vi "Configure Channel (TC Delta).vi"(0 "VISA resource name":refnum<visa-resource-name>, 1 "Reference Channel (0001)":string="0001", 5 "Channel (0001)":string="0001", 7 "Enable Channel (True)":bool=TRUE, 9 "Range and Span":T1={"Thermocouple Type (0 : R)"=0, "Enable Span (False)"=FALSE, "Lower Span (0.0)"=0.0, "Upper Span (1760.0)"=1760.0, "Bias (0)"=0.0} {"Thermocouple Type (0 : R)" items=["R", "S", "B", "K", "K-H", "E", "J", "T", "N", "W", "L", "U", "WRe3-25", "PLATINEL", "PR40-20", "KpvsAu7Fe", "NiNiMo", "WWRe26", "N14", "XK"]; "Bias (0)" min=-99999.9 max=99999.9 format="%.1f"; "Upper Span (1760.0)" min=-10000.0 max=10000.0 format="%#.1f"; "Lower Span (0.0)" min=-10000.0 max=10000.0 format="%#.1f"}, 11 "error in (no error)":errorcluster) -> (4 "VISA resource name out":refnum<visa-resource-name>, 6 "Channel":string, 15 "error out":errorcluster)   [LabVIEW 2020, in "Yokogawa GX Series.lvlib"]
doc: "Sets the input range as thermocouple.\n\nCommand: SRangeAI"
uses:
  <instrlib>/Yokogawa GX Series/Yokogawa GX Series.lvlib
  <instrlib>/Yokogawa GX Series/Private/TC Range.vi
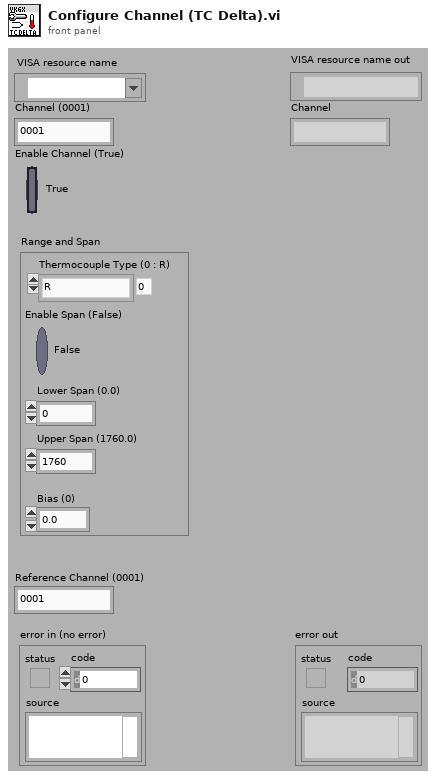
[diagram p1: front panel]
types:
  T1 = cluster{"Thermocouple Type (0 : R)":i32, "Enable Span (False)":bool, "Lower Span (0.0)":dbl, "Upper Span (1760.0)":dbl, "Bias (0)":dbl}
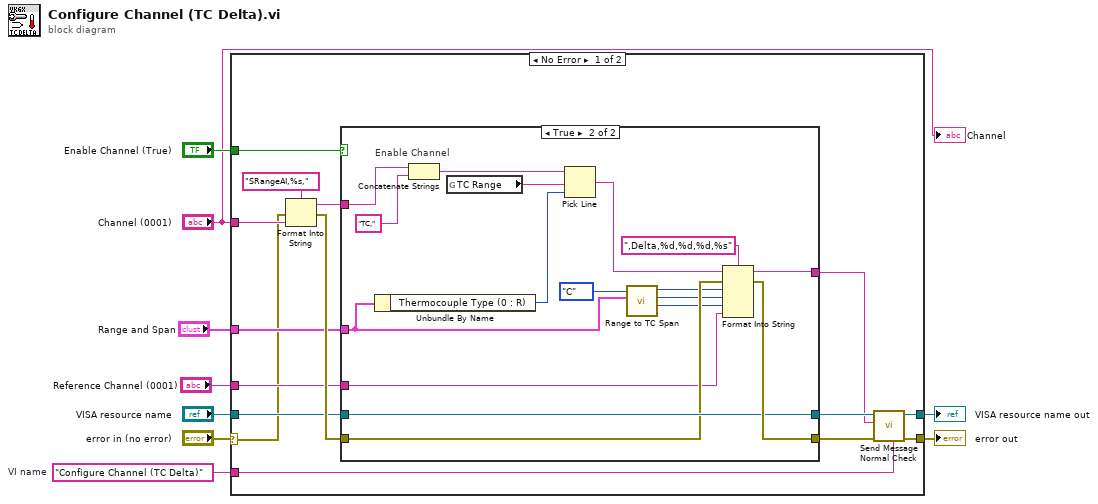
[diagram p0: block diagram]
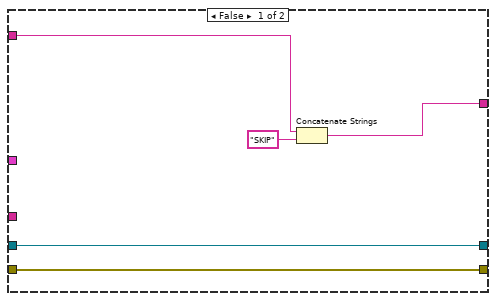
[diagram p2: hidden frame]
diagram:
  w4 = "Configure Channel (TC Delta)"  # VI name
  n1 = case shown="No Error" "error in (no error)" {
    selector: "error in (no error)" -> [w10 w47]
    tunnel: "Enable Channel (True)" -> [w21 _]
    tunnel: "VISA resource name" -> [w20 w48]
    tunnel: "Range and Span" -> [w19 _]
    tunnel: [w16 w48] -> w6
    tunnel: [w15 w47] -> w5
    tunnel: w4 -> [w14 _]
    tunnel: "Reference Channel (0001)" -> [w12 _]
    tunnel: "Channel (0001)" -> [w11 _]
    frame No Error {
      n2 = Format Into String(format string="SRangeAI,%s,", error in=w10, w11) -> (resulting string=w22:string, error out=w23:errorcluster)  [unwired: 1 in]
      n3 = case shown="True" w21 {
        tunnel: w23 -> [w26 w37]
        tunnel: [w26 w45] -> w17
        tunnel: w22 -> [w29 w40]
        tunnel: [w28 w43] -> w13
        tunnel: w20 -> [w25 w38]
        tunnel: [w25 w38] -> w18
        tunnel: w19 -> [_ w34]
        tunnel: w12 -> [_ w36]
        frame False {
          n4 = Concatenate Strings(w29, "SKIP") -> (w28:string)
        }
        frame True {
          # "Enable Channel"
          n5 = Unbundle By Name(w34) -> ("Thermocouple Type (0 : R)"=w39:i32)
          n6 = Concatenate Strings(w40, "TC,") -> (w42:string)
          n7 = global read "TC Range.vi" "TC Range"() -> (w30:string)
          n8 = Pick Line(string ("")=w42, multi-line string=w30, line index=w39) -> (output string=w44:string)
          n9 = call <instrlib>:"Range to TC Span.vi"("Range and Span"=w34, "Temp. Unit (0: C)"=enum16{"C", "F"}."C") -> ("Bias"=w31:i32, "Upper Span"=w32:i32, "Lower Span"=w33:i32)  [unwired: 7 in]
          n10 = Format Into String(format string=",Delta,%d,%d,%d,%s", initial string=w44, error in=w37, w33, w32, w31, w36) -> (resulting string=w43:string, error out=w45:errorcluster)
        }
      }
      n11 = call <instrlib>:"Send Message Normal Check.vi"("Source (\"\")"=w14, "error in (no error)"=w17, "Send Message (\"\")"=w13, "VISA resource name"=w18) -> ("error out"=w15:errorcluster, "VISA resource name out"=w16:refnum<visa-resource-name>)  [unwired: 2 in, 4 out]
    }
    frame Error {
    }
  }
  "error out" <- w5
  "VISA resource name out" <- w6
  "Channel" <- "Channel (0001)"
